vi "HumanGetDeviceReference.vi"() -> (1 "Aux Joy":T1, 3 "Driver Joy":T1)   [LabVIEW 2020]
uses:
  <vilib>/Rock Robotics/WPI/Joystick/WPI_JoystickDevRef.ctl
  <vilib>/Rock Robotics/WPI/Joystick/WPI_JoystickDeviceEnum.ctl
  <vilib>/Rock Robotics/WPI/Utilities/WPI_GetSetVariantRefNum.vi
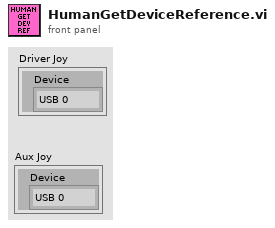
[diagram p1: front panel]
types:
  T1 = typedef "WPI_JoystickDevRef.ctl" = cluster{"Device":T2}
  T2 = typedef "WPI_JoystickDeviceEnum.ctl" = enum16{"USB 0", "USB 1", "USB 2", "USB 3", "USB 4", "USB 5"}
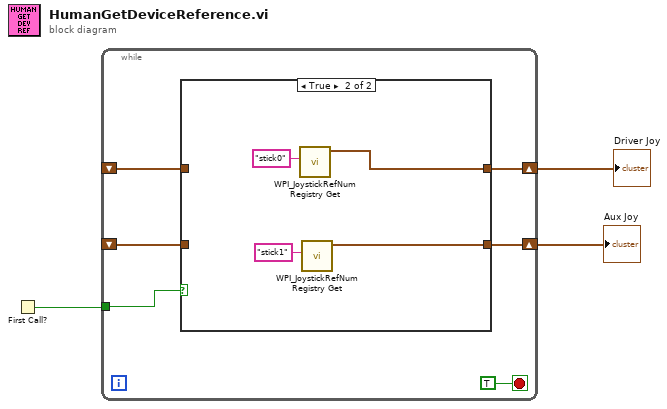
[diagram p0: block diagram]
diagram:
  n1 = First Call?() -> (First Call?: T/F=w1:bool)
  n2 = while {
    shift-right: [w7] -> w3
    shift-left: _ -> [w5]
    shift-right: [w6] -> w2
    shift-left: _ -> [w4]
    tunnel: w1 -> [w8]
    stop <- TRUE stop-if-true
    n3 = case shown="True" w8 {
      tunnel: [w11 w13] -> w7
      tunnel: [w10 w12] -> w6
      tunnel: w5 -> [w11 _]
      tunnel: w4 -> [w10 _]
      frame False {
      }
      frame True {
        n4 = call <vilib>:"WPI_JoystickRefNum Registry Get.vi"("refnum name"="stick0") -> ("JoystickDevRef"=w13:T1)  [unwired: 9 in, 1 out]
        n5 = call <vilib>:"WPI_JoystickRefNum Registry Get.vi"("refnum name"="stick1") -> ("JoystickDevRef"=w12:T1)  [unwired: 9 in, 1 out]
      }
    }
  }
  "Aux Joy" <- w2
  "Driver Joy" <- w3
